vi "Grant Pin Access.vi"(7 "Use External Browser? (F)":bool, 8 "error in (no error)":errorcluster, 10 "Request token":string, 11 "Authorize URL":string="https://api.twitter.com/oauth/authenticate") -> (0 "error out":errorcluster, 1 "Timeout?":bool, 2 "Pin":string)   [LabVIEW 2011, in "i3-oauth.lvlib"]
doc: "Opens an embedded or external browser, allowing the user to provide the PIN required for authentication."
uses:
  i3-oauth.lvlib
  <vilib>/Platform/browser.llb/Open URL in Default Browser (string).vi
panel:
  in  "Done":bool
  in  "Enter Pin Code Here":string
  in  "WebBrowser":refnum<k7>(container)
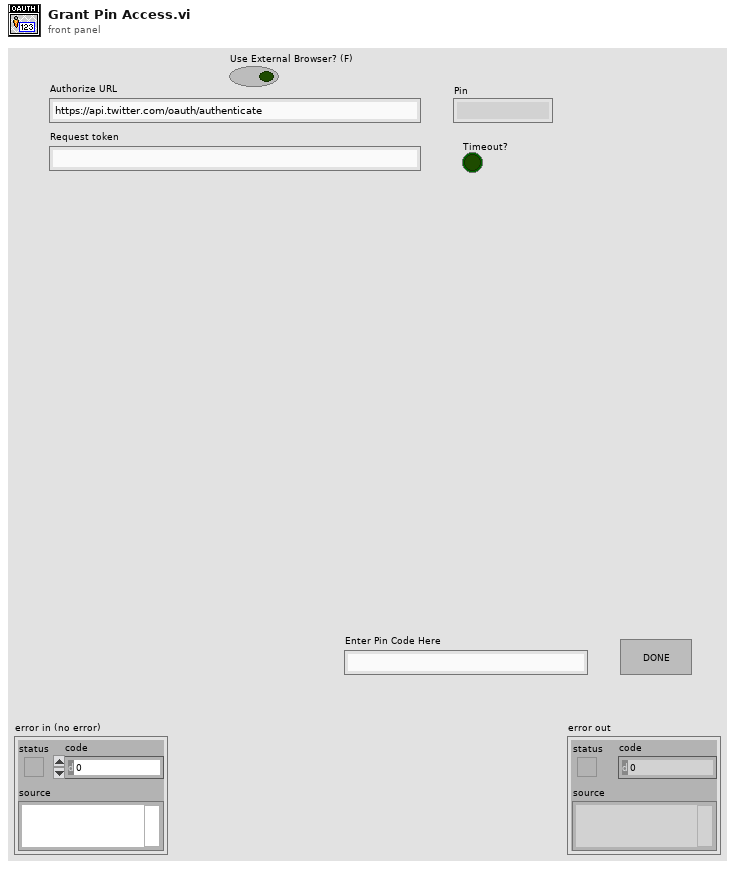
[diagram p1: front panel]
types:
  T1 = enum32{"Invalid", "Standard", "Closed", "Hidden", "Minimized", "Maximized"}
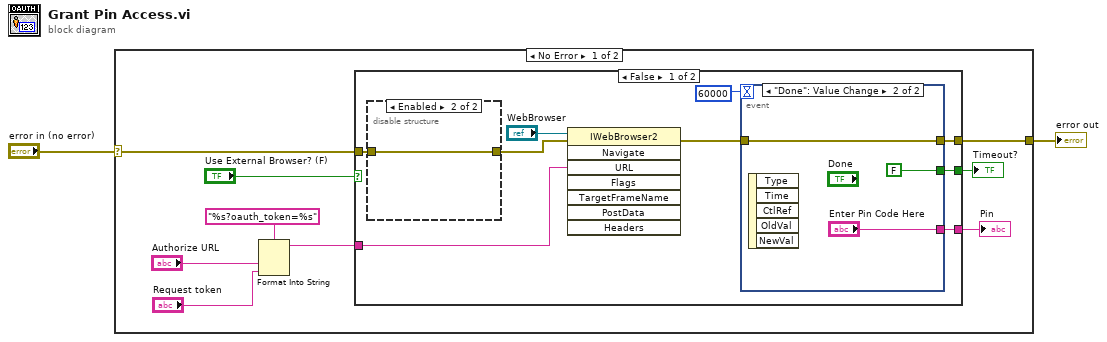
[diagram p0: block diagram]
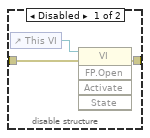
[diagram p2: hidden frame]
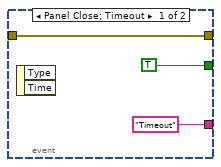
[diagram p3: hidden frame]
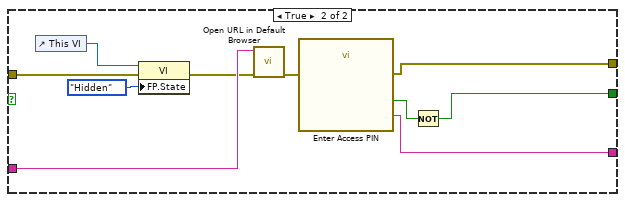
[diagram p4: hidden frame]
diagram:
  n1 = case shown="No Error" "error in (no error)" {
    selector: "error in (no error)" -> [w7 w41]
    tunnel: [w4 w41] -> w1
    frame No Error {
      n2 = Format Into String(format string="%s?oauth_token=%s", "Authorize URL", "Request token") -> (resulting string=w8:string)  [unwired: 2 in, 1 out]
      n3 = case shown="False" "Use External Browser? (F)" {
        tunnel: w8 -> [w19 w35]
        tunnel: w7 -> [w18 w34]
        tunnel: [w14 w38] -> w6
        tunnel: [w13 w37] -> w5
        tunnel: [w12 w40] -> w4
        frame False {
          n4 = disable-structure shown="Enabled" {
            disable-tunnel: w18 -> [w22 w24]
            disable-tunnel: [w21 w24] -> w17
            frame Disabled {
              n5 = control-ref of="This VI"() -> (w23:refnum<vi>)
              n6 = invoke class="VI" method="FP.Open"(reference=w23, error in=w22) -> (error out=w21:errorcluster)  [unwired: 3 in, 4 out]
            }
            frame Enabled {
            }
          }
          n7 = invoke class="IWebBrowser2" method="Navigate"(reference="WebBrowser", error in=w17, "URL"=w19) -> (error out=w15:errorcluster)  [unwired: 5 in, 7 out]
          n8 = event shown="[1] \"Done\": Value Change" {
            selector: _ -> [_ _]
            dyn-events: _ -> [_ _]
            timeout: 60000 -> [_ _]
            tunnel: w15 -> [w25 w28]
            tunnel: ["Timeout" ("Pin") "Enter Pin Code Here"] -> w14
            tunnel: [TRUE FALSE] -> w13
            tunnel: [w25 w28] -> w12
            event Panel Close; Timeout {
              n9 = event-data() -> ()  [unwired: 1 in, 2 out]
            }
            event "Done": Value Change {
              n10 = event-data() -> ()  [unwired: 1 in, 5 out]
            }
          }
        }
        frame True {
          n11 = control-ref of="This VI"() -> (w32:refnum<vi>)
          n12 = property class="VI"(reference=w32, error in=w34, "FP.State"=T1."Hidden" ("Front Panel Window:State")) -> (error out=w33:errorcluster)  [unwired: 1 out]
          n13 = call-poly <vilib>:"Open URL in Default Browser.vi"("error in (no error)"=w33, "URL"=w35) -> ("error out"=w36:errorcluster)  [unwired: 4 in, 1 out]
          n14 = call "Enter Access PIN"("error in (no error)"=w36) -> ("Enter Pin Here"=w38:string, "OK"=w39:bool, "error out"=w40:errorcluster)  [unwired: 16 in]
          n15 = Not(x=w39) -> (.not. x?=w37:bool)
        }
      }
      "Pin" <- w6
      "Timeout?" <- w5
    }
    frame Error {
    }
  }
  "error out" <- w1
